vi "stutusindicator.vi"(9 "String":string, 10 "Boolean":bool) -> (1 "?":bool, 2 "?":string, 3 "?":bool)   [LabVIEW 2018, in "LibInstrumentStatus.lvlib"]
uses:
  LibInstrumentStatus.lvlib
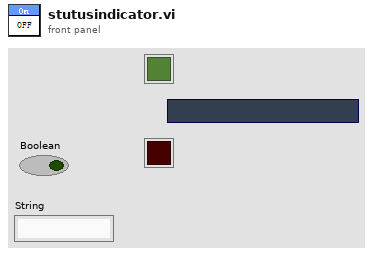
[diagram p1: front panel]
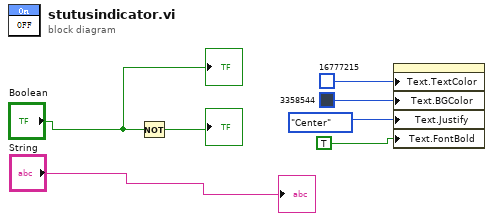
[diagram p0: block diagram]
diagram:
  n1 = Not(x="Boolean") -> (.not. x?=→"?":bool)
  n2 = property class="Str"("Text.TextColor"=u32 16777215, "Text.BGColor"=u32 3358544, "Text.Justify"=enum16{"Left", "Center", "Right"}."Center" ("Text.Justification"), "Text.FontBold"=TRUE ("Text.Font:Bold")) -> ()  [unwired: 2 in, 2 out]
  "?" <- "Boolean"
  "?" <- "String"
